vi "Piston Heater Interlock Configuration.vi"(8 "error in (no error)":errorcluster, 11 "cRIO-CO2 in":refnum<class "cRIO-CO2.lvclass">) -> (0 "error out":errorcluster, 2 "Interlock Chain":refnum<class "Interlock Chain.lvclass">, 3 "cRIO-CO2 out":refnum<class "cRIO-CO2.lvclass">)   [LabVIEW 2015, in "cRIO-Carbondioxide.lvlib" / "cRIO-CO2.lvlib" / "cRIO-CO2.lvclass"]
uses:
  cRIO-CO2.lvclass
  Interlocks/Interlock Chain/Interlock Chain.lvclass
  Interlocks/Interlock/Interlock.lvclass
  Interlocks/Interlock DBL/Range/Interlock Range.lvclass
  Interlocks/Interlock Bool/Interlock Bool.lvclass
  Interlocks/Interlock Bool/Interlock Bool.lvclass/Interlock Bool.ctl
  Interlocks/Interlock DBL/Range/Interlock Range.lvclass/Interlock Range.ctl
  Interlocks/Interlock Chain/Interlock Chain.lvclass/Interlock Chain.ctl
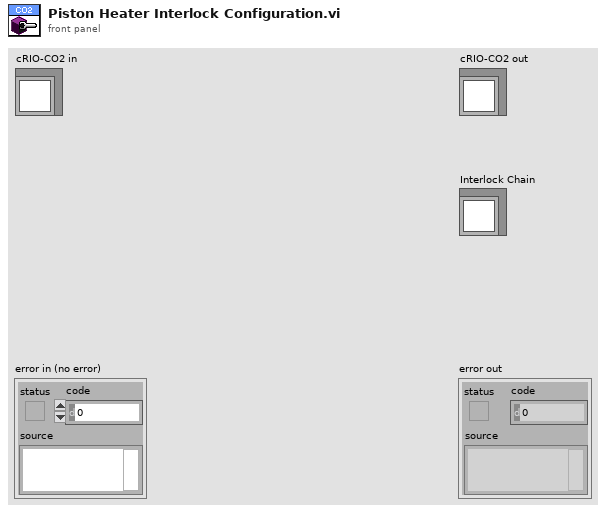
[diagram p1: front panel]
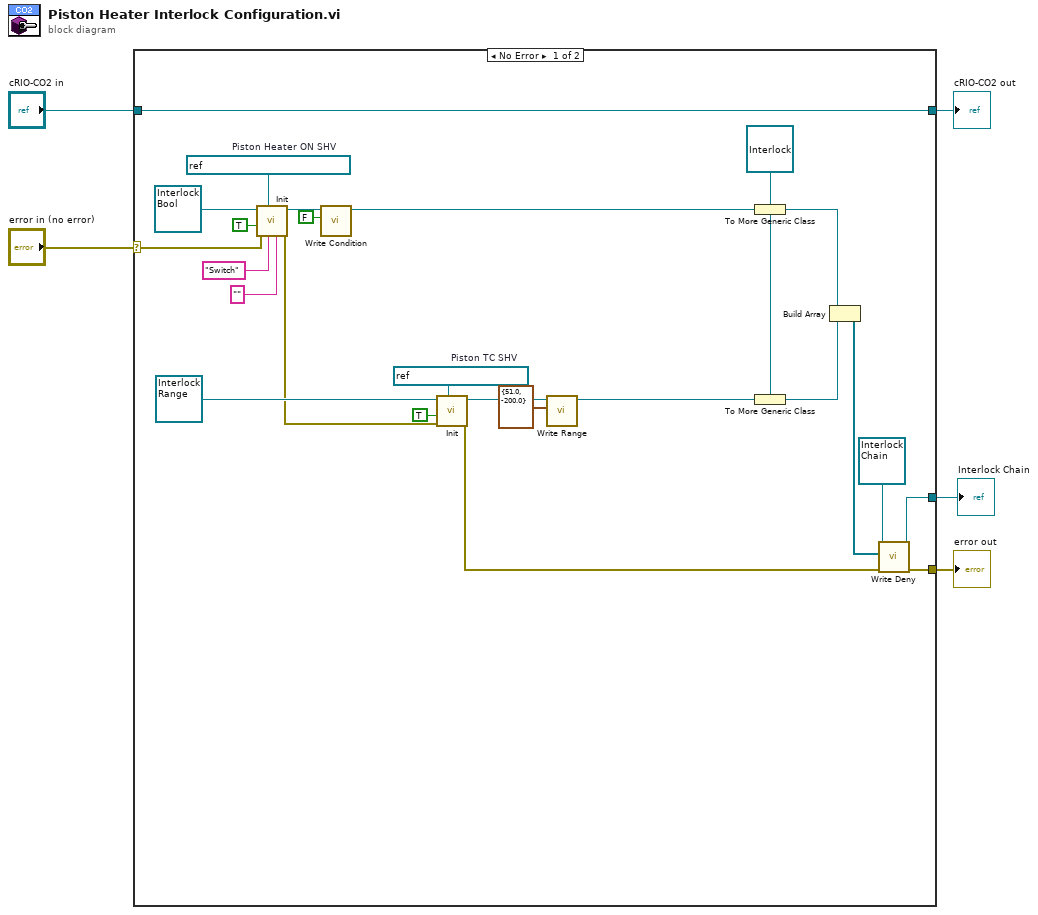
[diagram p0: block diagram]
diagram:
  n1 = case shown="No Error" "error in (no error)" {
    selector: "error in (no error)" -> [w20 w32]
    tunnel: [w13 w32] -> w4
    tunnel: [w30 w31] -> w2
    tunnel: "cRIO-CO2 in" -> [w30 w31]
    tunnel: [w11 _] -> w1
    frame No Error {
      w22 = refnum<k21> "ni.var.psp://10.2.0.20/AMS Gas SHV/Heaters/Piston Heater ON"  # Piston Heater ON SHV
      w27 = refnum<k21> "ni.var.psp://10.2.0.20/AMS Gas SHV/Gauges/Piston TC"  # Piston TC SHV
      w17 = refnum<class "Interlock.lvclass"> refnum ("Interlock.lvclass")
      n2 = call-dynamic "Init.vi"("Interlock message (\" -> Interlock!\")"="" ("Interlock message (\" -> Interlock!\")"), "Name (SHV Name if empty)"="Switch", "SHV"=w22, "error in (no error)"=w20, "Stop Self on IL? (T)"=TRUE, "Interlock in"=refnum<class "Interlock Bool.lvclass"> refnum ("Interlock Bool.lvclass")) -> ("error out"=w8:errorcluster, "Interlock out"=w23:refnum<class "Interlock Bool.lvclass">)  [unwired: 4 in]
      n3 = call "Write Condition.vi"("Interlock Condition"=FALSE, "Interlock Bool in"=w23) -> ("Interlock Bool out"=w18:refnum<class "Interlock Bool.lvclass">)  [unwired: 8 in, 1 out]
      n4 = call-dynamic "Init.vi"("SHV"=w27, "error in (no error)"=w8, "Stop Self on IL? (T)"=TRUE, "Interlock in"=refnum<class "Interlock Range.lvclass"> refnum ("Interlock DBL.lvclass")) -> ("error out"=w14:errorcluster, "Interlock out"=w28:refnum<class "Interlock Range.lvclass">)  [unwired: 6 in]
      n5 = call "Write Range.vi"("Range"=cluster{"Upper Limit":dbl, "Lower Limit":dbl} {"Upper Limit"=51.0, "Lower Limit"=-200.0}, "Interlock Bool in"=w28) -> ("Interlock Bool out"=w25:refnum<class "Interlock Range.lvclass">)  [unwired: 8 in, 1 out]
      n6 = To More Generic Class(target class=w17, reference=w18) -> (generic class reference=w16:refnum<class "Interlock.lvclass">)
      n7 = To More Generic Class(target class=w17, reference=w25) -> (generic class reference=w9:refnum<class "Interlock.lvclass">)
      n8 = Build Array(w16, w9) -> (w12:refnum<class "Interlock.lvclass">[])
      n9 = call "Write Deny.vi"("error in (no error)"=w14, "Deny"=w12, "Interlock Chain in"=refnum<class "Interlock Chain.lvclass"> refnum) -> ("error out"=w13:errorcluster, "Interlock Chain out"=w11:refnum<class "Interlock Chain.lvclass">)  [unwired: 7 in]
    }
    frame Error {
    }
  }
  "error out" <- w4
  "cRIO-CO2 out" <- w2
  "Interlock Chain" <- w1
